vi "ADO Recordset self design.vi"(0 "ADODB._Recordset In":refnum<k7>, 2 "Fields":i32, 3 "Values":string, 5 "error in (no error)":errorcluster, 7 "Command Text":string) -> (14 "ADODB._Recordset Out":refnum<k7>, 19 "error out":errorcluster)   [LabVIEW 2018]
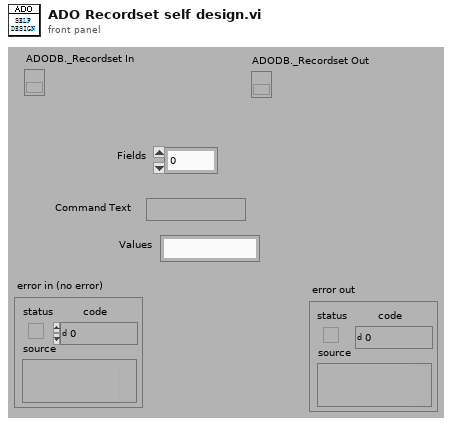
[diagram p1: front panel]
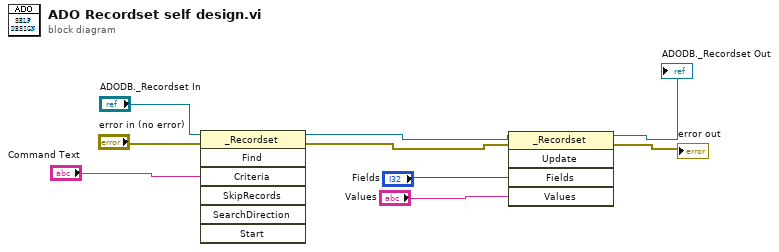
[diagram p0: block diagram]
diagram:
  n1 = invoke class="_Recordset" method="Find"(reference="ADODB._Recordset In", error in="error in (no error)", "Criteria"="Command Text") -> (reference out=w6:refnum<k7>, error out=w5:errorcluster)  [unwired: 4 in, 5 out]
  n2 = invoke class="_Recordset" method="Update"(reference=w6, error in=w5, "Fields"="Fields", "Values"="Values") -> (reference out=→"ADODB._Recordset Out":refnum<k7>, error out=→"error out":errorcluster)  [unwired: 1 in, 3 out]
